vi "Get CBOR Structure Value.vi"(8 "error in (no error)":errorcluster, 11 "CBOR Hex":string) -> (0 "error out":errorcluster, 1 "Structure Value":u8, 3 "Remaining Data":string)   [LabVIEW 2020, in "CBOR.lvlib"]
uses:
  CBOR.lvlib
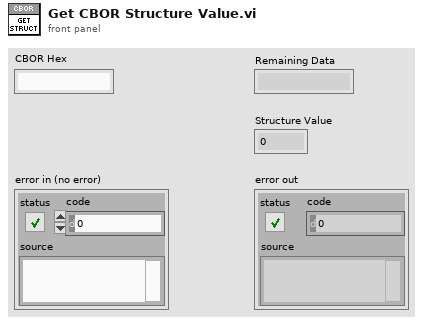
[diagram p1: front panel]
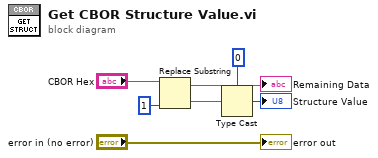
[diagram p0: block diagram]
diagram:
  n1 = Replace Substring(2:1 ("length (len. of substring)"), 5:"CBOR Hex") -> (0:w3:string, 1:→"Remaining Data":string)  [unwired: 2 in]
  n2 = Type Cast(type=u8 0, x=w3) -> (*(type *) &x=→"Structure Value":u8)
  "error out" <- "error in (no error)"
